vi "PRBS64 Core.vi"(11 "current value":u64) -> (3 "next value":u64)   [LabVIEW 2023, in "Aurora64b66b Utilities FPGA.lvlib"]
uses:
  Aurora64b66b Utilities FPGA.lvlib
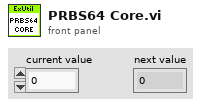
[diagram p1: front panel]
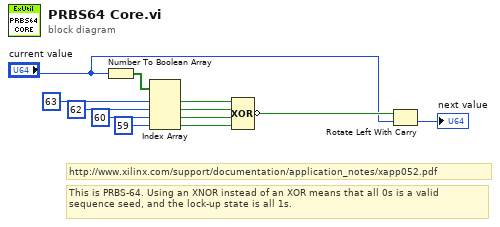
[diagram p0: block diagram]
diagram:
  # "This is PRBS-64. Using an XNOR instead of an XOR means that all 0s is a valid sequence seed, and the lock-up state is all 1s."
  # "http://www.xilinx.com/support/documentation/application_notes/xapp052.pdf"
  n1 = Number To Boolean Array(number="current value") -> (Boolean array=w7:bool[])
  n2 = Index Array(array=w7, index #1=63 ("index"), index #2=62 ("index"), index #3=60 ("index"), index #4=59 ("index")) -> (element #1=w9:bool, element #2=w8:bool, element #3=w10:bool, element #4=w11:bool)
  n3 = Compound Arithmetic op=XOR(w9, w8, w10, w11) -> (invert w12:bool)
  n4 = Rotate Left With Carry(2:"current value", 3:w12) -> (0:→"next value":u64)  [unwired: 1 out]
